vi "Agilent VNA Set Start and Stop Frequencies.vi"(6 "Channel":i8=1 min=1 max=99 step=1, 7 "Agilent VNA":T1, 8 "error in (no error)":errorcluster, 9 "CW? (f)":bool, 10 "Start/Stop Freqs, MHz":cluster{"Fstart":dbl, "Fstop":dbl}, 11 "VISA Resource Name":refnum<visa-resource-name>) -> (0 "error out":errorcluster, 3 "dup VISA Resource Name":refnum<visa-resource-name>)   [LabVIEW 2011]
doc: "This VI for the HP 8753B is used to read the number of stimulus points."
uses:
  TypeDefs/Agilent VNA Instrument Info.ctl
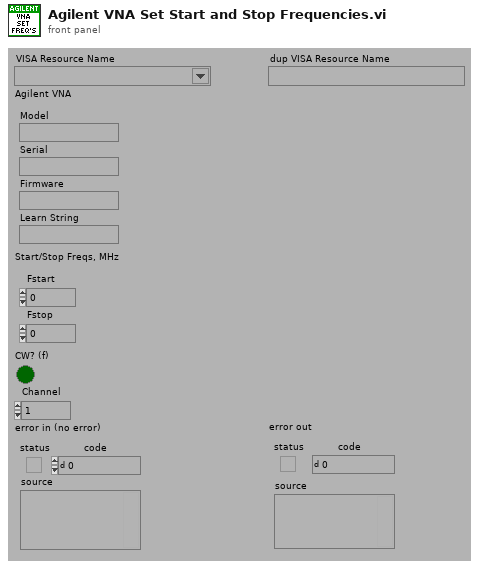
[diagram p1: front panel]
types:
  T1 = typedef "Agilent VNA Instrument Info.ctl" = cluster{"Model":string, "Serial":string, "Firmware":string, "Learn String":string}
  T2 = typedef "Agilent VNA Model.ctl" = enum16{"Not Supported", "8510X", "8719X", "8720X", "8722X", "8753X", "ENA", "PNA", "Field Fox"}
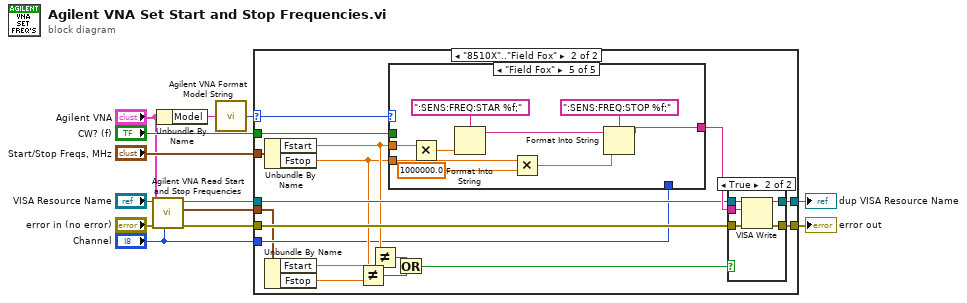
[diagram p0: block diagram]
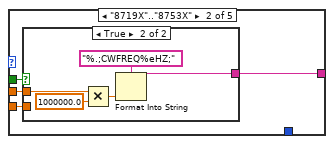
[diagram p4: hidden frame]
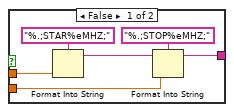
[diagram p5: hidden frame]
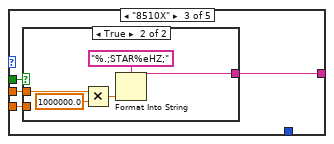
[diagram p6: hidden frame]
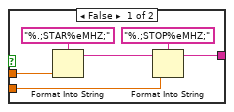
[diagram p7: hidden frame]
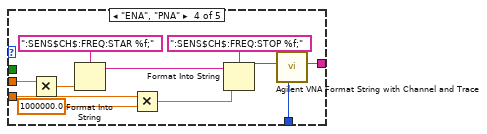
[diagram p8: hidden frame]
diagram:
  n1 = call "Agilent VNA Read Start and Stop Frequencies.vi"("Channel"="Channel", "Agilent VNA"="Agilent VNA", "error in (no error)"="error in (no error)", "VISA Resource Name"="VISA Resource Name") -> ("error out"=w7:errorcluster, "Start/Stop Freqs, MHz"=w5:cluster{"Fstart":dbl, "Fstop":dbl}, "dup VISA Resource Name"=w6:refnum<visa-resource-name>)  [unwired: 5 out]
  n2 = Unbundle By Name("Agilent VNA") -> ("Model"=w3:string)
  n3 = call "Agilent VNA Format Model String.vi"("Model"=w3) -> ("Model"=w1:T2)
  n4 = case shown="\"8510X\"..\"Field Fox\"" w1 {
    selector: w1 -> [_ w17]
    tunnel: [w14 w32] -> w13
    tunnel: [w15 w31] -> w12
    tunnel: "Start/Stop Freqs, MHz" -> [_ w30]
    tunnel: "CW? (f)" -> [_ w28]
    tunnel: w7 -> [w15 w27]
    tunnel: w6 -> [w14 w26]
    tunnel: w5 -> [_ w16]
    tunnel: "Channel" -> [_ w18]
    frame "Not Supported" {
    }
    frame "8510X".."Field Fox" {
      n5 = Unbundle By Name(w30) -> ("Fstart"=w25:dbl, "Fstop"=w23:dbl)
      n6 = Unbundle By Name(w16) -> ("Fstart"=w24:dbl, "Fstop"=w22:dbl)
      n7 = Not Equal?(x=w23, y=w22) -> (x != y?=w20:bool)
      n8 = Not Equal?(x=w25, y=w24) -> (x != y?=w21:bool)
      n9 = case shown="\"Field Fox\"" w17 {
        tunnel: [_ w36 w51 w64 w74] -> w29
        tunnel: w28 -> [_ w35 w50 _ _]
        tunnel: w25 -> [_ w34 w49 w70 w79]
        tunnel: w23 -> [_ w33 w48 w68 w77]
        tunnel: w18 -> [_ _ _ w63 _]
        frame "Not Supported" {
        }
        frame "8719X".."8753X" {
          n10 = case shown="True" w35 {
            tunnel: w34 -> [w40 w46]
            tunnel: w33 -> [w38 _]
            tunnel: [w37 w44] -> w36
            frame False {
              n11 = Format Into String(format string="%.;STAR%eMHZ;", w40) -> (resulting string=w39:string)  [unwired: 2 in, 1 out]
              n12 = Format Into String(format string="%.;STOP%eMHZ;", initial string=w39, w38) -> (resulting string=w37:string)  [unwired: 1 in, 1 out]
            }
            frame True {
              n13 = Multiply(x=w46, y=1000000.0) -> (x*y=w45:dbl)
              n14 = Format Into String(format string="%.;CWFREQ%eHZ;", w45) -> (resulting string=w44:string)  [unwired: 2 in, 1 out]
            }
          }
        }
        frame "8510X" {
          n15 = case shown="True" w50 {
            tunnel: w49 -> [w55 w61]
            tunnel: w48 -> [w53 _]
            tunnel: [w52 w59] -> w51
            frame False {
              n16 = Format Into String(format string="%.;STAR%eMHZ;", w55) -> (resulting string=w54:string)  [unwired: 2 in, 1 out]
              n17 = Format Into String(format string="%.;STOP%eMHZ;", initial string=w54, w53) -> (resulting string=w52:string)  [unwired: 1 in, 1 out]
            }
            frame True {
              n18 = Multiply(x=w61, y=1000000.0) -> (x*y=w60:dbl)
              n19 = Format Into String(format string="%.;STAR%eHZ;", w60) -> (resulting string=w59:string)  [unwired: 2 in, 1 out]
            }
          }
        }
        frame "ENA", "PNA" {
          w66 = 1000000.0 ("y")
          n20 = Multiply(x=w70, y=w66) -> (x*y=w69:dbl)
          n21 = Format Into String(format string=":SENS$CH$:FREQ:STAR %f;", w69) -> (resulting string=w71:string)  [unwired: 2 in, 1 out]
          n22 = Multiply(x=w68, y=w66) -> (x*y=w67:dbl)
          n23 = Format Into String(format string=":SENS$CH$:FREQ:STOP %f;", initial string=w71, w67) -> (resulting string=w65:string)  [unwired: 1 in, 1 out]
          n24 = call "Agilent VNA Format String with Channel and Trace.vi"("Channel"=w63, "String"=w65) -> ("String Out"=w64:string)  [unwired: 1 in, 6 out]
        }
        frame "Field Fox" {
          w75 = 1000000.0 ("y")
          n25 = Multiply(x=w79, y=w75) -> (x*y=w78:dbl)
          n26 = Format Into String(format string=":SENS:FREQ:STAR %f;", w78) -> (resulting string=w80:string)  [unwired: 2 in, 1 out]
          n27 = Multiply(x=w77, y=w75) -> (x*y=w76:dbl)
          n28 = Format Into String(format string=":SENS:FREQ:STOP %f;", initial string=w80, w76) -> (resulting string=w74:string)  [unwired: 1 in, 1 out]
        }
      }
      n29 = Or(x=w21, y=w20) -> (x .or. y?=w19:bool)
      n30 = case shown="True" w19 {
        tunnel: [w84 w89] -> w32
        tunnel: [w83 w88] -> w31
        tunnel: w29 -> [_ w87]
        tunnel: w27 -> [w83 w86]
        tunnel: w26 -> [w84 w85]
        frame False {
        }
        frame True {
          n31 = VISA Write(VISA resource name=w85, write buffer=w87, error in (no error)=w86) -> (VISA resource name out=w89:refnum<visa-resource-name>, error out=w88:errorcluster)  [unwired: 1 out]
        }
      }
    }
  }
  "dup VISA Resource Name" <- w13
  "error out" <- w12
